vi "update_logging_waveform_array.vi"(8 "error in (no error)":errorcluster caption="错误输入（无错误）", 10 "new waveform array":waveform(dbl)[](array[waveform]) caption="新波形数组", 11 "original waveform array":waveform(dbl)[](array[waveform]) caption="原波形数组") -> (0 "error out":errorcluster caption="错误输出", 1 "max duration":dbl caption="最大时长", 2 "min duration":dbl caption="最小时长", 3 "updated wavefrom array":waveform(dbl)[](array[waveform]) caption="更新后波形数组")   [LabVIEW 2015]
uses:
  <vilib>/Waveform/WDTOps.llb/WDT Index Channel DBL.vi
  <vilib>/Waveform/WDTOps.llb/WDT Append Waveforms DBL.vi
  <vilib>/Waveform/WDTOps.llb/WDT Waveform Duration DBL.vi
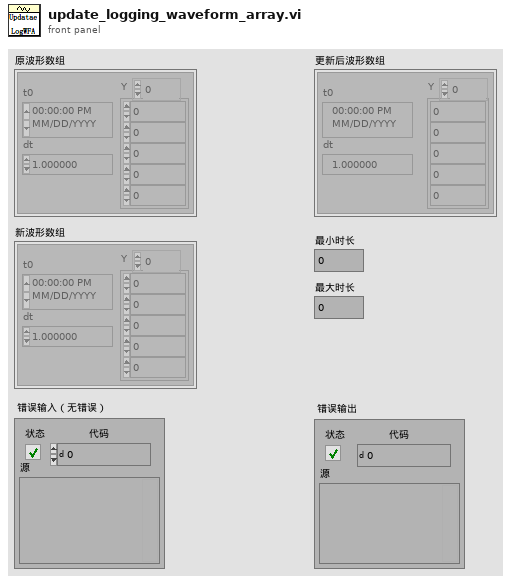
[diagram p1: front panel]
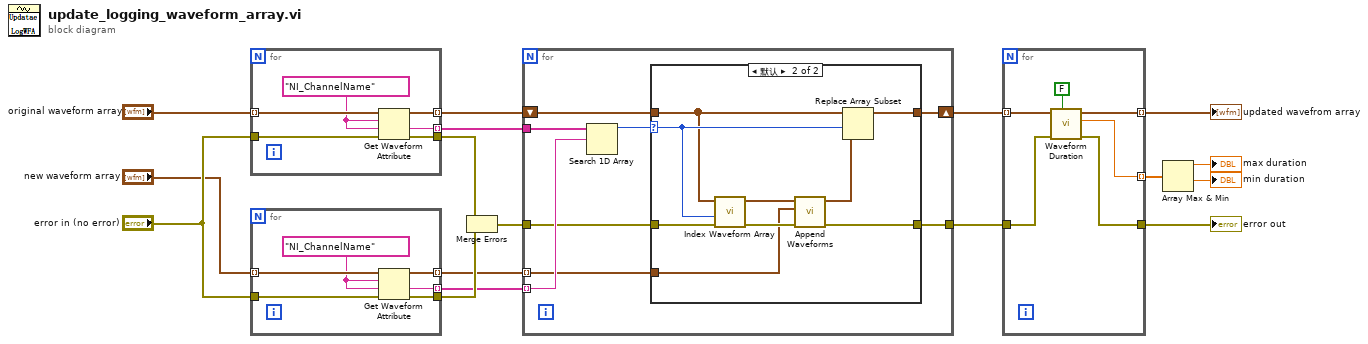
[diagram p0: block diagram]
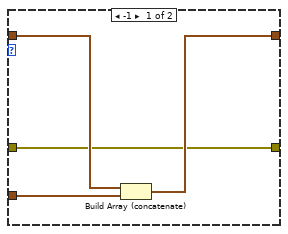
[diagram p2: hidden frame]
diagram:
  n1 = for {
    tunnel: "original waveform array" -> [w23] mode=indexing
    tunnel: "error in (no error)" -> [w22]
    tunnel: [w20] -> w15 mode=indexing
    tunnel: [w19] -> w14 mode=indexing
    tunnel: [w18] -> w12
    w21 = "NI_ChannelName" ("名称")
    n2 = Get Waveform Attribute(4:w22, 5:w21, 6:w21, 7:w23) -> (0:w18:errorcluster, 1:w20:string, 3:w19:waveform(dbl))  [unwired: 1 out]
  }
  n3 = for {
    tunnel: "new waveform array" -> [w29] mode=indexing
    tunnel: "error in (no error)" -> [w28]
    tunnel: [w26] -> w11 mode=indexing
    tunnel: [w25] -> w10 mode=indexing
    tunnel: [w24] -> w13
    w27 = "NI_ChannelName" ("名称")
    n4 = Get Waveform Attribute(4:w28, 5:w27, 6:w27, 7:w29) -> (0:w24:errorcluster, 1:w26:string, 3:w25:waveform(dbl))  [unwired: 1 out]
  }
  n5 = Merge Errors(w12, w13) -> (w9:errorcluster)
  n6 = for {
    tunnel: w15 -> [w37]
    tunnel: w11 -> [w36] mode=indexing
    tunnel: w10 -> [w33] mode=indexing
    shift-right: [w31] -> w8
    shift-left: w14 -> [w32]
    tunnel: w9 -> [w34]
    tunnel: [w30] -> w6
    n7 = Search 1D Array(1D array=w37, element=w36) -> (index of element=w35:i32)  [unwired: 1 in]
    n8 = case shown="默认" w35 {
      selector: w35 -> [_ w46]
      tunnel: w32 -> [w41 w42]
      tunnel: w34 -> [w38 w48]
      tunnel: w33 -> [w40 w47]
      tunnel: [w39 w44] -> w31
      tunnel: [w38 w43] -> w30
      frame -1 {
        n9 = Build Array (concatenate)(w41, w40) -> (w39:waveform(dbl)[])
      }
      frame Default {
        n10 = call-poly <vilib>:"Index Waveform Array.vi"("error in (no error)"=w48, "index"=w46, "waveform array"=w42) -> ("error out"=w49:errorcluster, "waveform"=w50:waveform(dbl))  [unwired: 7 in]
        n11 = call-poly <vilib>:"Append Waveforms.vi"("error in (no error)"=w49, "waveform B"=w47, "waveform A"=w50) -> ("error out"=w43:errorcluster, "waveform out"=w45:waveform(dbl))  [unwired: 7 in]
        n12 = Replace Array Subset(array=w42, new element=w45, index=w46) -> (w44:waveform(dbl)[])
      }
    }
  }
  n13 = for {
    tunnel: w8 -> [w56] mode=indexing
    tunnel: [w55] -> w7 mode=indexing
    tunnel: w6 -> [w54]
    tunnel: [w53] -> w5
    tunnel: [w52] -> w3 mode=indexing
    n14 = call-poly <vilib>:"Waveform Duration.vi"("open interval? (T)"=FALSE, "error in (no error)"=w54, "waveform in"=w56) -> ("error out"=w53:errorcluster, "duration"=w52:dbl, "waveform out"=w55:waveform(dbl))  [unwired: 6 in]
  }
  "error out" <- w5
  "updated wavefrom array" <- w7
  n15 = Array Max & Min(array=w3) -> (max value=→"max duration":dbl, min value=→"min duration":dbl)  [unwired: 2 out]
